vi "Celsius Temperature Simulator.vi"(11 "에러 입력(에러 없음)":errorcluster) -> (4 "온도":dbl, 15 "에러 출력":errorcluster)   [LabVIEW 2018]
doc: "20도와 30도 사이의 임의의 시뮬레이션 온도를 생성합니다."
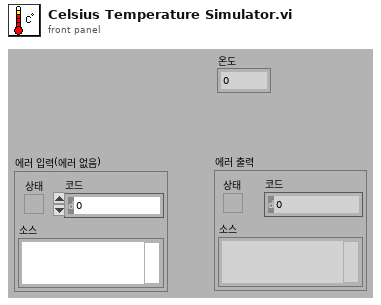
[diagram p1: front panel]
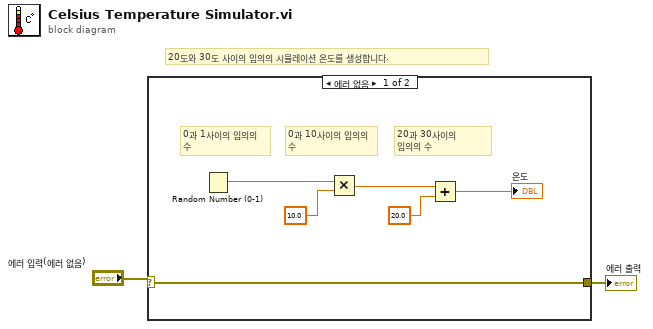
[diagram p0: block diagram]
diagram:
  # "20도와 30도 사이의 임의의 시뮬레이션 온도를 생성합니다."
  n1 = case shown="에러 없음" "에러 입력(에러 없음)" {
    selector: "에러 입력(에러 없음)" -> [w3 w9]
    tunnel: [w3 w9] -> w1
    frame No Error {
      # "20과 30사이의 임의의 수"
      # "0과 10사이의 임의의 수"
      # "0과 1사이의 임의의 수"
      n2 = Random Number (0-1)() -> (number: 0 to 1=w8:dbl)
      n3 = Multiply(x=w8, y=10.0) -> (x*y=w6:dbl)
      n4 = Add(x=w6, y=20.0) -> (x+y=→"온도":dbl)
    }
    frame Error {
    }
  }
  "에러 출력" <- w1
